vi "Resize Table 1D.vi"(11 "1D Table":refnum<vi>) -> ()   [LabVIEW 2016]
uses:
  <vilib>/addons/Software Calibration Management/XControls/TBL1D.xctl
panel:
  out "Y Size":i32
  in  "X Size":i32=2 min=2
  in  "Cancel Button":bool
  in  "OK Button":bool
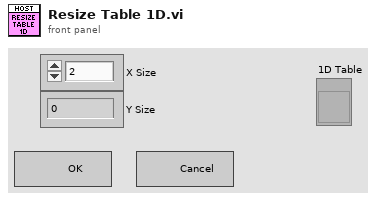
[diagram p1: front panel]
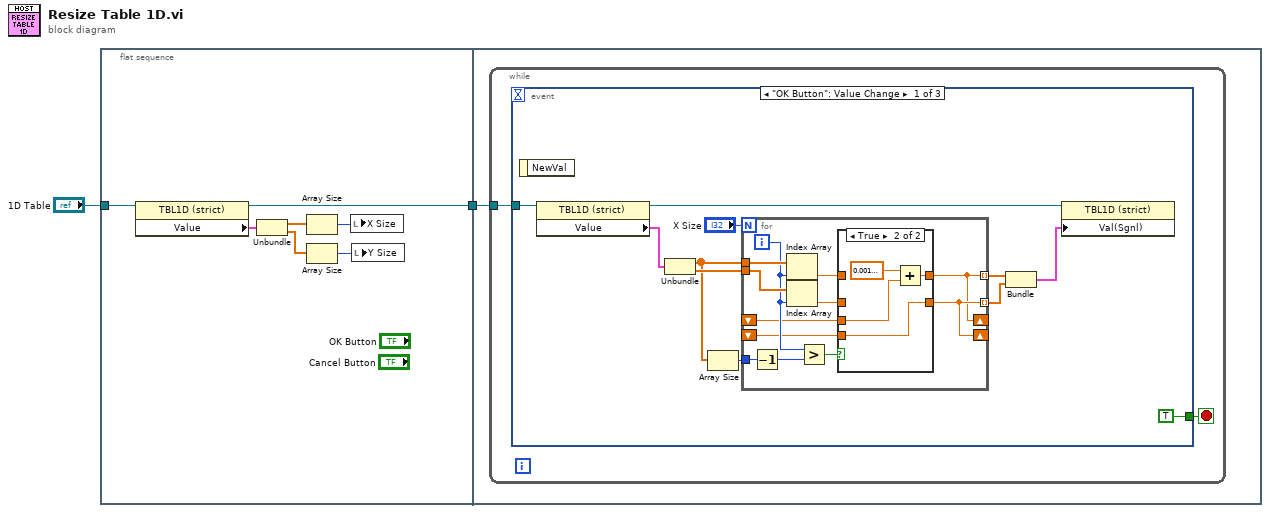
[diagram p0: block diagram]
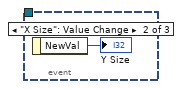
[diagram p3: hidden frame]
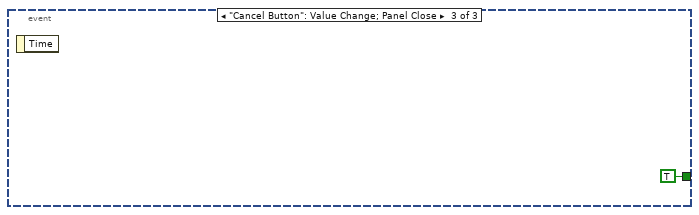
[diagram p4: hidden frame]
diagram:
  n1 = flat-sequence {
    tunnel: "1D Table" -> [w5]
    tunnel: [w3] -> w1
    tunnel: w1 -> [w10]
    frame #0 {
      n2 = property class="TBL1D (strict)"(reference=w5) -> (reference out=w3:refnum<vi>, "Value"=w4:cluster{"X":sgl[], "Y":sgl[]})  [unwired: 1 in, 1 out]
      n3 = Unbundle(w4) -> ("X"=w8:sgl[], "Y"=w7:sgl[])
      n4 = Array Size(array=w8) -> (size(s)=w9:i32)
      n5 = Array Size(array=w7) -> (size(s)=w6:i32)
      n6 = local write "X Size"(w9) -> ()
      n7 = local write "Y Size"(w6) -> ()
    }
    frame #1 {
      n8 = while {
        tunnel: w10 -> [w11]
        stop <- w12 stop-if-true
        n9 = event shown="[0] \"OK Button\": Value Change" {
          selector: _ -> [_ _ _]
          dyn-events: _ -> [_ _ _]
          timeout: _ -> [_ _ _]
          tunnel: [TRUE _ TRUE] -> w12
          tunnel: w11 -> [w22 _ _]
          event "OK Button": Value Change {
            n10 = event-data() -> ()  [unwired: 1 in, 1 out]
            n11 = property class="TBL1D (strict)"(reference=w22) -> (reference out=w21:refnum<vi>, "Value"=w20:cluster{"X":sgl[], "Y":sgl[]})  [unwired: 1 in, 1 out]
            n12 = Unbundle(w20) -> ("X"=w17:sgl[], "Y"=w19:sgl[])
            n13 = Array Size(array=w17) -> (size(s)=w16:i32)
            n14 = for {
              N: "X Size" -> [_]
              tunnel: w17 -> [w35]
              tunnel: w19 -> [w34]
              tunnel: w16 -> [w29]
              tunnel: [w25] -> w15 mode=indexing
              tunnel: [w27] -> w14 mode=indexing
              shift-right: [w27] -> _
              shift-left: _ -> [w26]
              shift-right: [w25] -> _
              shift-left: _ -> [w24]
              i -> [w33]
              n15 = Decrement(x=w29) -> (x-1=w28:i32)
              n16 = Index Array(array=w35, index=w33) -> (element=w31:sgl)
              n17 = Index Array(array=w34, index=w33) -> (element=w30:sgl)
              n18 = Greater?(x=w33, y=w28) -> (0:w32:bool)
              n19 = case shown="True" w32 {
                tunnel: [w37 w39] -> w25
                tunnel: w31 -> [w37 _]
                tunnel: w30 -> [w36 _]
                tunnel: [w36 w41] -> w27
                tunnel: w26 -> [_ w41]
                tunnel: w24 -> [_ w40]
                frame False {
                }
                frame True {
                  n20 = Add(x=sgl 0.001, y=w40) -> (x+y=w39:sgl)
                }
              }
            }
            n21 = Bundle(w15, w14) -> (w13:cluster{sgl[], sgl[]})  [unwired: 1 in]
            n22 = property class="TBL1D (strict)"(reference=w21, "Val(Sgnl)"=w13) -> ()  [unwired: 1 in, 2 out]
          }
          event "X Size": Value Change {
            n23 = event-data() -> ("NewVal"=→"Y Size":i32)  [unwired: 1 in]
          }
          event "Cancel Button": Value Change; Panel Close {
            n24 = event-data() -> ()  [unwired: 1 in, 1 out]
          }
        }
      }
    }
  }
